vi "SDCP SMF Transmitter and Receiver - Logger Loop.vi"(3 "error in (no error)":errorcluster, 4 "Trace File Path in":path) -> (0 "error out":errorcluster, 1 "Trace File Path out":path)   [LabVIEW 2020]
uses:
  <vilib>/Utility/file.llb/Write Delimited Spreadsheet (string).vi
  Global Stop.vi
panel:
  out "queue empty":bool
  out "# elements in queue":i32
  out "size(s)":i32
  out "save interval (ms)":u32
  out "Save to file":bool
  out "Log data":cluster{"Record":string[]}[](array[cluster])
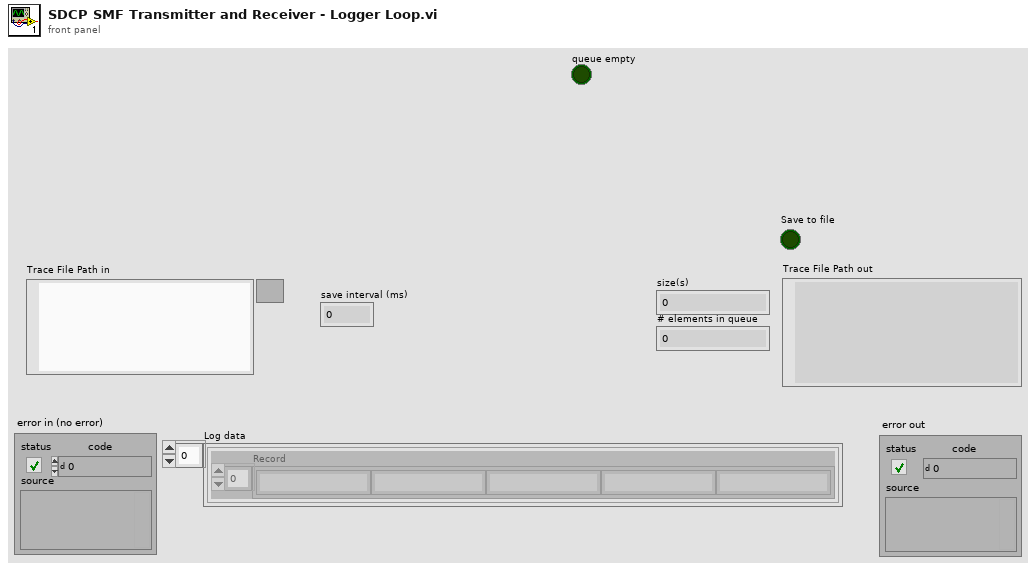
[diagram p1: front panel]
types:
  T1 = typedef "SDCP SMF Receiver and Transmitter - Notifier and Queues.ctl" = cluster{"Trace Queue":refnum<queue>, "Tx - Log Table Queue":refnum<queue>, "Tx - User Queue":refnum<queue>, "Rx - Log Table Queue":refnum<queue>, "Rx - User Queue":refnum<queue>, "Log status Notifier":refnum<notifier>, "Plot Queue":refnum<queue>}
  T2 = enum16{"open", "replace", "create", "open or create", "replace or create", "replace or create with confirmation"}
  T3 = typedef "SDCP SMF logger - SMF with timestamp.ctl" = cluster{"Bytes":u8[], "Checksum":bool, "Time (ms)":u32, "Tx/Rx":string}
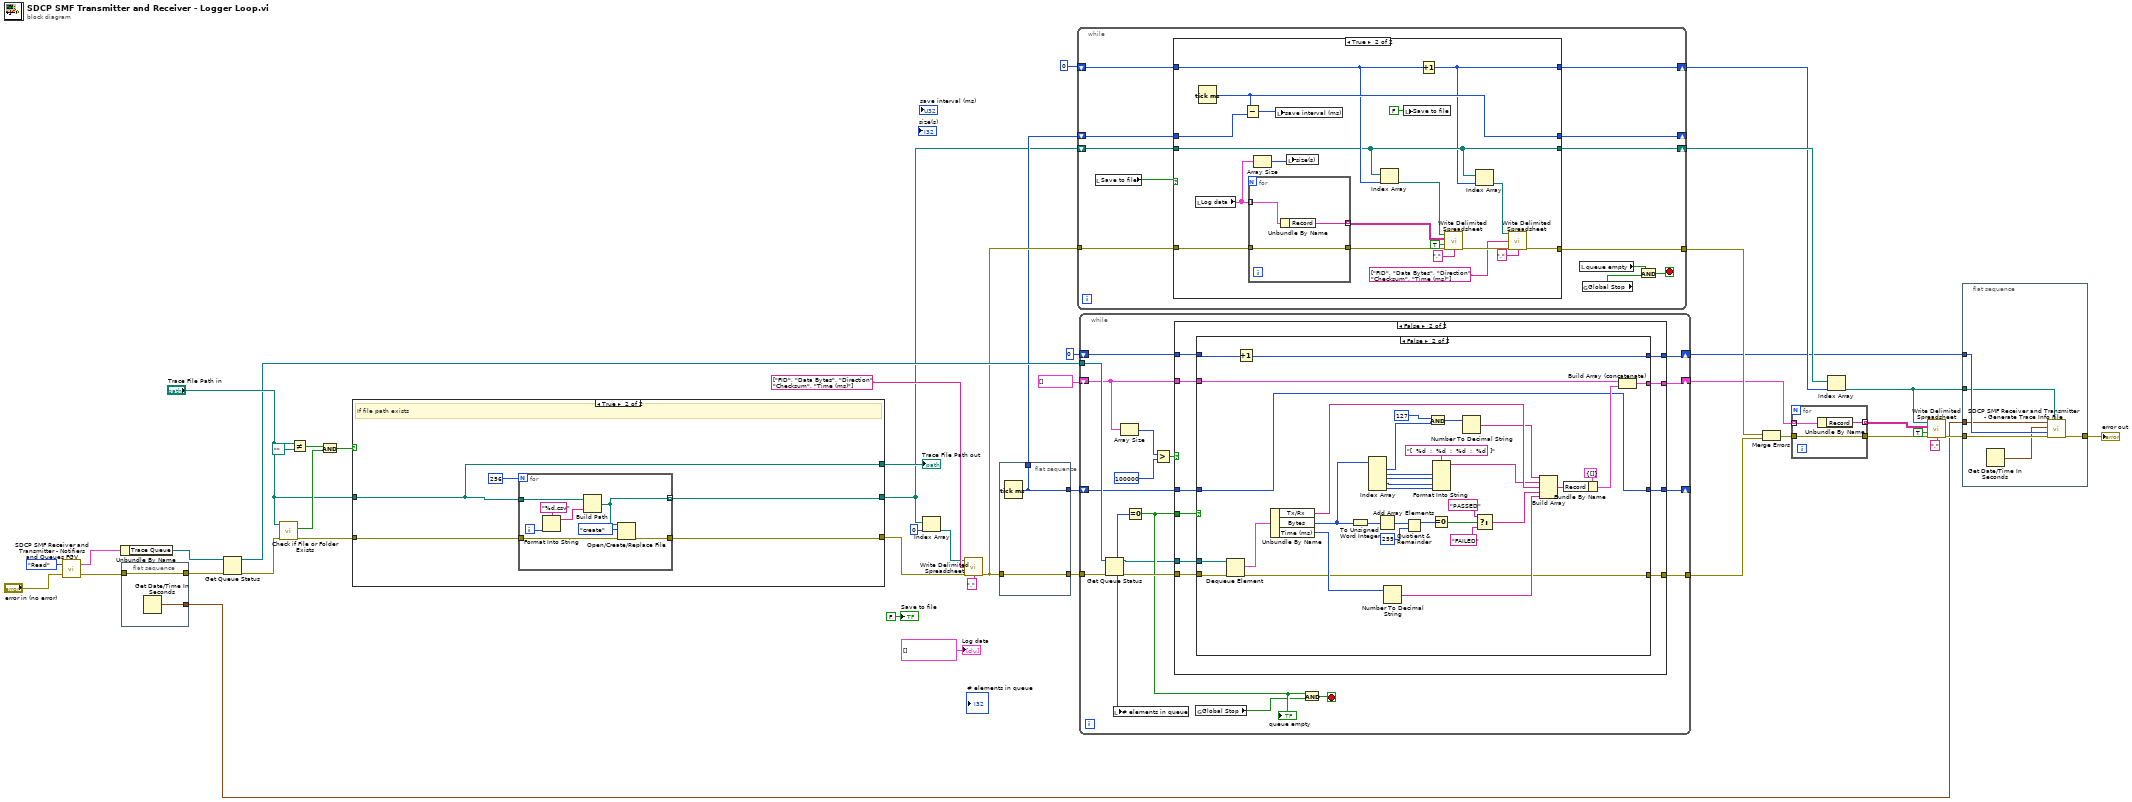
[diagram p0: block diagram]
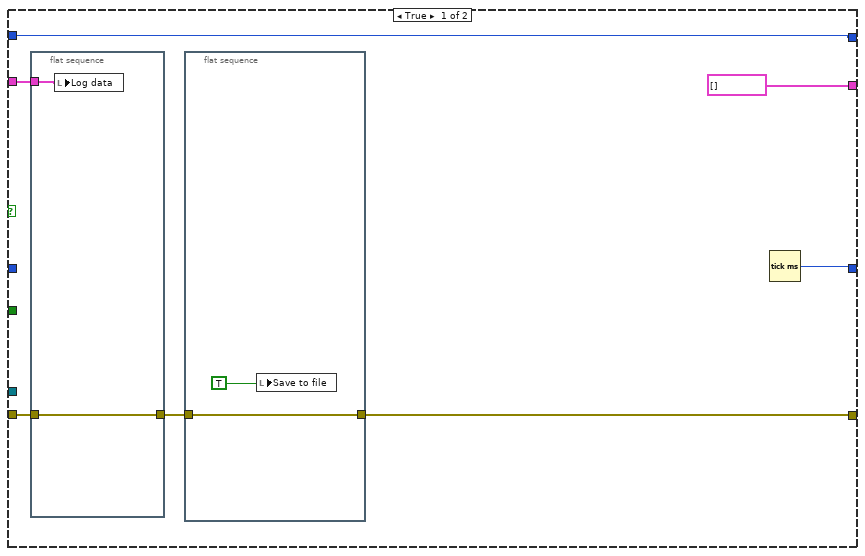
[diagram p3: hidden frame]
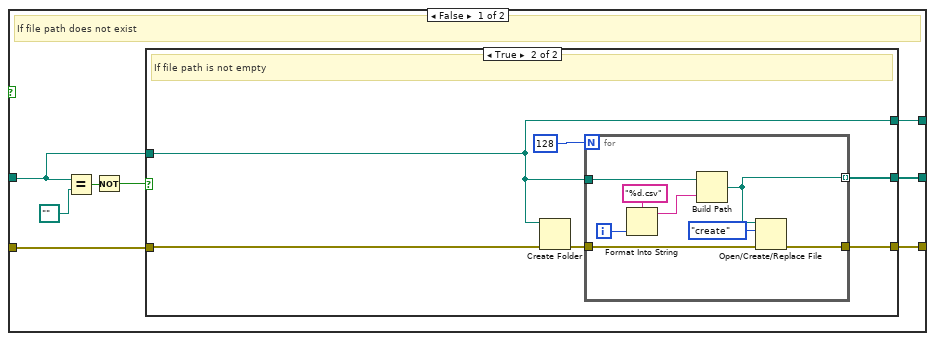
[diagram p5: hidden frame]
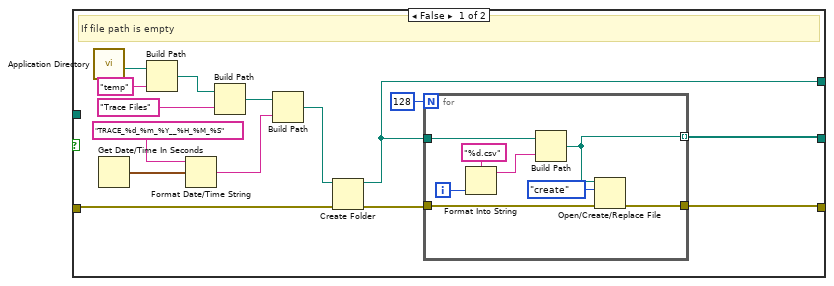
[diagram p6: hidden frame]
diagram:
  n1 = call "SDCP SMF Receiver and Transmitter - Notifiers and Queues FGV.vi"("error in (no error)"="error in (no error)", "Command"=enum16{"Initialize", "Read", "Deinitialize"}."Read") -> ("error out"=w3:errorcluster, "Output"=w11:T1)
  n2 = Unbundle By Name(w11) -> ("Trace Queue"=w10:refnum<queue>)
  n3 = flat-sequence {
    tunnel: w3 -> [w47]
    tunnel: [w47] -> w2
    tunnel: [w46] -> w1
    frame #0 {
      n4 = Get Date/Time In Seconds() -> (seconds since 1Jan1904=w46:timestamp)
    }
  }
  n5 = Get Queue Status(queue=w10, error in (no error)=w2) -> (queue out=w35:refnum<queue>, error out=w37:errorcluster)  [unwired: 1 in, 6 out]
  n6 = call <vilib>:"Check if File or Folder Exists.vi"("error in (no error)"=w37, "path"="Trace File Path in") -> ("error out"=w45:errorcluster, "file or folder exists?"=w40:bool)  [unwired: 7 in, 1 out]
  n7 = Not Equal?(x="Trace File Path in", y=path "") -> (x != y?=w39:bool)
  n8 = And(x=w39, y=w40) -> (x .and. y?=w41:bool)
  n9 = case shown="True" w41 {
    tunnel: w45 -> [w55 w95]
    tunnel: "Trace File Path in" -> [w53 w93]
    tunnel: [w54 w94] -> w44
    tunnel: [w49 w96] -> w24
    tunnel: [w48 w93] -> w25
    frame False {
      # "If file path does not exist"
      n10 = Equal?(x=w53, y=path "") -> (x = y?=w51:bool)
      n11 = Not(x=w51) -> (.not. x?=w50:bool)
      n12 = case shown="True" w50 {
        tunnel: w55 -> [w62 w84]
        tunnel: w53 -> [_ w79]
        tunnel: [w58 w81] -> w54
        tunnel: [w59 w80] -> w49
        tunnel: [w57 w79] -> w48
        frame False {
          # "If file path is empty"
          n13 = call <vilib>:"Application Directory.vi"() -> ("Application Directory"=w70:path)
          n14 = Get Date/Time In Seconds() -> (seconds since 1Jan1904=w65:timestamp)
          n15 = Build Path(base path=w70, name or relative path="temp") -> (appended path=w68:path)
          n16 = Format Date/Time String(time format string (%c)="TRACE_%d_%m_%Y__%H_%M_%S", seconds (now)=w65) -> (date/time string=w63:string)  [unwired: 1 in]
          n17 = Build Path(base path=w68, name or relative path="Trace Files") -> (appended path=w66:path)
          n18 = Build Path(base path=w66, name or relative path=w63) -> (appended path=w61:path)
          n19 = Create Folder(path (use dialog)=w61, error in=w62) -> (created path=w57:path, error out=w60:errorcluster)  [unwired: 1 in, 1 out]
          n20 = for {
            N: 128 -> [_]
            tunnel: w57 -> [w78]
            tunnel: w60 -> [w74]
            tunnel: [w72] -> w58
            tunnel: [w71] -> w59 mode=indexing
            i -> [w76]
            n21 = Format Into String(format string="%d.csv", w76) -> (resulting string=w75:string)  [unwired: 2 in, 1 out]
            n22 = Build Path(base path=w78, name or relative path=w75) -> (appended path=w71:path)
            n23 = Open/Create/Replace File(file path (use dialog)=w71, error in=w74, operation (0:open)=T2."create") -> (error out=w72:errorcluster)  [unwired: 3 in, 2 out]
          }
        }
        frame True {
          # "If file path is not empty"
          n24 = Create Folder(path (use dialog)=w79, error in=w84) -> (error out=w83:errorcluster)  [unwired: 1 in, 2 out]
          n25 = for {
            N: 128 -> [_]
            tunnel: w79 -> [w92]
            tunnel: w83 -> [w88]
            tunnel: [w86] -> w81
            tunnel: [w85] -> w80 mode=indexing
            i -> [w90]
            n26 = Format Into String(format string="%d.csv", w90) -> (resulting string=w89:string)  [unwired: 2 in, 1 out]
            n27 = Build Path(base path=w92, name or relative path=w89) -> (appended path=w85:path)
            n28 = Open/Create/Replace File(file path (use dialog)=w85, error in=w88, operation (0:open)=T2."create") -> (error out=w86:errorcluster)  [unwired: 3 in, 2 out]
          }
        }
      }
    }
    frame True {
      # "If file path exists"
      n29 = for {
        N: 256 -> [_]
        tunnel: w93 -> [w105]
        tunnel: w95 -> [w101]
        tunnel: [w99] -> w94
        tunnel: [w98] -> w96 mode=indexing
        i -> [w103]
        n30 = Format Into String(format string="%d.csv", w103) -> (resulting string=w102:string)  [unwired: 2 in, 1 out]
        n31 = Build Path(base path=w105, name or relative path=w102) -> (appended path=w98:path)
        n32 = Open/Create/Replace File(file path (use dialog)=w98, error in=w101, operation (0:open)=T2."create") -> (error out=w99:errorcluster)  [unwired: 3 in, 2 out]
      }
    }
  }
  "Trace File Path out" <- w25
  n33 = Index Array(array=w24, index=0) -> (element=w23:path)
  n34 = call-poly <vilib>:"Write Delimited Spreadsheet.vi"("file path (dialog if empty)"=w23, "1D data"=string[] ["FID", "Data Bytes", "Direction", "Checksum", "Time (ms)"], "error in (no error)"=w44, "delimiter (\\t)"="," ("delimiter (\\t)")) -> ("error out"=w31:errorcluster)  [unwired: 10 in, 1 out]
  n35 = flat-sequence {
    tunnel: w31 -> [w107]
    tunnel: [w107] -> w34
    tunnel: [w106] -> w33
    tunnel: [w106] -> w30
    frame #0 {
      n36 = Tick Count (ms)() -> (millisecond timer value=w106:u32)
    }
  }
  n37 = while {
    tunnel: w31 -> [w118]
    shift-right: [w114] -> _
    shift-left: w30 -> [w115]
    tunnel: [w116] -> w28
    shift-right: [w113] -> w20
    shift-left: w24 -> [w117]
    shift-right: [w111] -> w13
    shift-left: 0 -> [w112]
    stop <- w108 stop-if-true
    n38 = local read "Save to file"() -> (w119:bool)
    n39 = case shown="True" w119 {
      tunnel: w118 -> [w122 w143]
      tunnel: w117 -> [w121 w128]
      tunnel: [w122 w125] -> w116
      tunnel: w115 -> [w123 w139]
      tunnel: [w123 w138] -> w114
      tunnel: [w121 w128] -> w113
      tunnel: w112 -> [w120 w133]
      tunnel: [w120 w127] -> w111
      frame False {
      }
      frame True {
        n40 = local read "Log data"() -> (w136:cluster{"Record":string[]}[])
        n41 = Tick Count (ms)() -> (millisecond timer value=w138:u32)
        n42 = Subtract(x=w138, y=w139) -> (x-y=w135:u32)
        n43 = for {
          tunnel: w143 -> [w144]
          tunnel: w136 -> [w146] mode=indexing
          tunnel: [w145] -> w131 mode=indexing
          tunnel: [w144] -> w142
          n44 = Unbundle By Name(w146) -> ("Record"=w145:string[])
        }
        n45 = Array Size(array=w136) -> (size(s)=w134:i32)
        n46 = local write "save interval (ms)"(w135) -> ()
        n47 = local write "size(s)"(w134) -> ()
        n48 = Index Array(array=w128, index=w133) -> (element=w132:path)
        n49 = local write "Save to file"(FALSE ("Save to file")) -> ()
        n50 = Increment(x=w133) -> (x+1=w127:i32)
        n51 = call-poly <vilib>:"Write Delimited Spreadsheet.vi"("file path (dialog if empty)"=w132, "2D data"=w131, "append to file? (new file:F)"=TRUE, "error in (no error)"=w142, "delimiter (\\t)"="," ("delimiter (\\t)")) -> ("error out"=w130:errorcluster)  [unwired: 9 in, 1 out]
        n52 = Index Array(array=w128, index=w127) -> (element=w126:path)
        n53 = call-poly <vilib>:"Write Delimited Spreadsheet.vi"("file path (dialog if empty)"=w126, "1D data"=string[] ["FID", "Data Bytes", "Direction", "Checksum", "Time (ms)"], "error in (no error)"=w130, "delimiter (\\t)"="," ("delimiter (\\t)")) -> ("error out"=w125:errorcluster)  [unwired: 10 in, 1 out]
      }
    }
    n54 = local read "queue empty"() -> (w110:bool)
    n55 = global read "Global Stop.vi" "Global Stop"() -> (w109:bool)
    n56 = And(x=w110, y=w109) -> (x .and. y?=w108:bool)
  }
  n57 = while {
    tunnel: w34 -> [w164]
    tunnel: w35 -> [w163]
    shift-right: [w154] -> _
    shift-left: w33 -> [w155]
    shift-right: [w157] -> w16
    shift-left: cluster{"Record":string[]}[] [] -> [w152]
    tunnel: [w156] -> w29
    shift-right: [w147] -> w5
    shift-left: u32 0 -> [w148]
    stop <- w161 stop-if-true
    n58 = Get Queue Status(queue=w163, error in (no error)=w164) -> (queue out=w158:refnum<queue>, error out=w162:errorcluster, # elements in queue=w153:i32)  [unwired: 1 in, 5 out]
    n59 = local write "# elements in queue"(w153) -> ()
    n60 = Array Size(array=w152) -> (size(s)=w150:i32)
    n61 = Equal To 0?(x=w153) -> (x = 0?=w160:bool)
    "queue empty" <- w160
    n62 = Greater?(x=w150, y=100000) -> (0:w151:bool)
    n63 = case shown="False" w151 {
      tunnel: w162 -> [w168 w185]
      tunnel: w160 -> [_ w184]
      tunnel: w158 -> [_ w183]
      tunnel: w152 -> [w169 w182]
      tunnel: [cluster{"Record":string[]}[] [] w181] -> w157
      tunnel: [w166 w180] -> w156
      tunnel: w155 -> [_ w179]
      tunnel: [w170 w178] -> w154
      tunnel: w148 -> [w165 w177]
      tunnel: [w165 w176] -> w147
      frame True {
        n64 = flat-sequence {
          tunnel: w169 -> [w175]
          tunnel: w168 -> [w174]
          tunnel: [w174] -> w167
          frame #0 {
            n65 = local write "Log data"(w175) -> ()
          }
        }
        n66 = flat-sequence {
          tunnel: w167 -> [w172]
          tunnel: [w172] -> w166
          frame #0 {
            n67 = local write "Save to file"(TRUE ("Save to file")) -> ()
          }
        }
        n68 = Tick Count (ms)() -> (millisecond timer value=w170:u32)
      }
      frame False {
        n69 = case shown="False" w184 {
          tunnel: w185 -> [w188 w199]
          tunnel: w183 -> [_ w198]
          tunnel: w182 -> [w189 w196]
          tunnel: [w189 w194] -> w181
          tunnel: [w188 w193] -> w180
          tunnel: w179 -> [w187 w192]
          tunnel: [w187 w192] -> w178
          tunnel: w177 -> [w186 w191]
          tunnel: [w186 w190] -> w176
          frame True {
          }
          frame False {
            n70 = Dequeue Element(queue=w198, error in (no error)=w199) -> (element=w197:T3, error out=w193:errorcluster)  [unwired: 1 in, 2 out]
            n71 = Increment(x=w191) -> (x+1=w190:u32)
            n72 = Unbundle By Name(w197) -> ("Tx/Rx"=w207:string, "Bytes"=w218:u8[], "Time (ms)"=w208:u32)
            n73 = To Unsigned Word Integer(number=w218) -> (unsigned 16bit integer=w217:u16[])
            n74 = Index Array(array=w218) -> (element #1=w205:u8, element #2=w222:u8, element #3=w221:u8, element #4=w220:u8, element #5=w219:u8)  [unwired: 5 in]
            n75 = Add Array Elements(numeric array=w217) -> (sum=w216:u16)
            n76 = Number To Decimal String(number=w208) -> (decimal integer string=w210:string)  [unwired: 1 in]
            n77 = Quotient & Remainder(x=w216, y=u16 255) -> (x-y*floor(x/y)=w214:u16)  [unwired: 1 out]
            n78 = And(x=u8 127, y=w205) -> (x .and. y?=w203:u8)
            n79 = Format Into String(format string="[  %d  :  %d  :  %d  :  %d  ]", w222, w221, w220, w219) -> (resulting string=w206:string)  [unwired: 2 in, 1 out]
            n80 = Equal To 0?(x=w214) -> (x = 0?=w213:bool)
            n81 = Number To Decimal String(number=w203) -> (decimal integer string=w202:string)  [unwired: 1 in]
            n82 = Select(t="PASSED", s=w213, f="FAILED") -> (s? t:f=w209:string)
            n83 = Build Array(w202, w206, w207, w209, w210) -> (w200:string[])
            n84 = Bundle By Name(cluster=cluster{"Record":string[]} {"Record"=[]}, "Record"=w200) -> (w195:cluster{"Record":string[]})
            n85 = Build Array (concatenate)(w196, w195) -> (w194:cluster{"Record":string[]}[])
          }
        }
      }
    }
    n86 = global read "Global Stop.vi" "Global Stop"() -> (w159:bool)
    n87 = And(x=w160, y=w159) -> (x .and. y?=w161:bool)
  }
  n88 = Merge Errors(w28, w29) -> (w18:errorcluster)
  n89 = for {
    tunnel: w18 -> [w226]
    tunnel: [w226] -> w17
    tunnel: w16 -> [w225] mode=indexing
    tunnel: [w224] -> w15 mode=indexing
    n90 = Unbundle By Name(w225) -> ("Record"=w224:string[])
  }
  n91 = Index Array(array=w20, index=w13) -> (element=w4:path)
  n92 = call-poly <vilib>:"Write Delimited Spreadsheet.vi"("file path (dialog if empty)"=w4, "2D data"=w15, "append to file? (new file:F)"=TRUE, "error in (no error)"=w17, "delimiter (\\t)"="," ("delimiter (\\t)")) -> ("error out"=w8:errorcluster)  [unwired: 9 in, 1 out]
  n93 = flat-sequence {
    tunnel: w8 -> [w232]
    tunnel: [w231] -> w7
    tunnel: w5 -> [w230]
    tunnel: w4 -> [w228]
    tunnel: w1 -> [w227]
    frame #0 {
      n94 = Get Date/Time In Seconds() -> (seconds since 1Jan1904=w229:timestamp)
      n95 = call "SDCP SMF Receiver and Transmitter - Generate Trace Info File.vi"("Trace File Path"=w228, "error in (no error)"=w232, "Number of samples"=w230, "Stop Time"=w229, "Start Time"=w227) -> ("error out"=w231:errorcluster)  [unwired: 6 in]
    }
  }
  "error out" <- w7
  "Save to file" <- FALSE ("Save to file")
  "Log data" <- cluster{"Record":string[]}[] [] ("Log data")
